vi "Slope Sub VI.vi"(1 "Y2":dbl, 2 "X2":dbl, 3 "Y1":dbl, 4 "X1":dbl) -> (0 "Slope":dbl)   [LabVIEW 2012]
doc: "A VI that will calculate a slope value given two \"x\" inputs and two \"y\" inputs together with an output indicator.\n\nThis VI contains:\n\n4 Num Ctrl\n1 Num Ind"
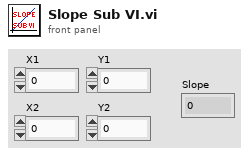
[diagram p1: front panel]
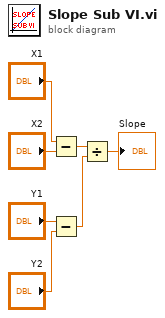
[diagram p0: block diagram]
diagram:
  n1 = Subtract(x="X1", y="X2") -> (x-y=w6:dbl)
  n2 = Subtract(x="Y1", y="Y2") -> (x-y=w5:dbl)
  n3 = Divide(x=w6, y=w5) -> (x/y=→"Slope":dbl)
